vi "Teleop.vi"(10 "Match Info":T1={"Autonomous Elapsed Seconds"=0.0, "TeleOp Elapsed Seconds"=0.0, "Disabled Elapsed Seconds"=0.0, "Visited Autonomous"=FALSE, "Visited TeleOp"=FALSE, "Visited Disabled"=FALSE, "Autonomous Settings"={"Autonomous Style"=enum."Independent", "VI Refnum"=refnum}}, 11 "Call Context":T2) -> ()   [LabVIEW 2014]
doc: "This VI is called for each TeleOp packet received from the DS where the robot is not disabled. It is often used to read from the joysticks and update I/O or to update setpoints for timed control loops. It should complete and return within 20 milliseconds or it may miss DS packets."
uses:
  <vilib>/Rock Robotics/WPI/DriverStation/WPI_DriverStationDerivedRobotMode.ctl
  <vilib>/Rock Robotics/WPI/DriverStation/WPI_DriverStationMatch Info.ctl
  <vilib>/Rock Robotics/WPI/Solenoid/WPI_SolenoidValue.ctl
  <vilib>/Rock Robotics/WPI/RobotDrive/WPI_RobotDriveGetSetRefNum.vi
  <vilib>/Rock Robotics/WPI/Joystick/WPI_JoystickGetSetRefNum.vi
  <vilib>/Rock Robotics/Network Tables/SD Write Boolean Array.vi
  <vilib>/Rock Robotics/Network Tables/SD Write Numeric Array.vi
  <vilib>/Rock Robotics/WPI/Compressor/WPI_CompressorGetSetRefNum.vi
  <vilib>/Rock Robotics/WPI/Solenoid/WPI_SolenoidSetEnum.vi
  hhVI/hhVI.lvlib
panel:
  out "Compressor Running":bool
  out "Enabled":bool
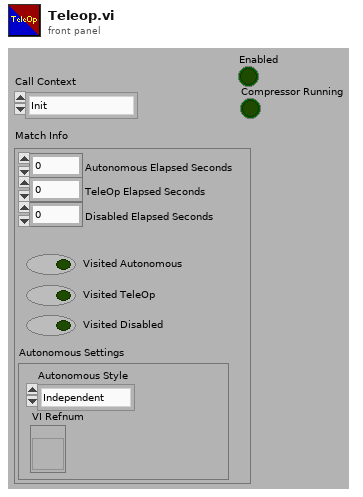
[diagram p1: front panel]
types:
  T1 = typedef "WPI_DriverStationMatch Info.ctl" = cluster{"Autonomous Elapsed Seconds":dbl, "TeleOp Elapsed Seconds":dbl, "Disabled Elapsed Seconds":dbl, "Visited Autonomous":bool, "Visited TeleOp":bool, "Visited Disabled":bool, "Autonomous Settings":cluster{"Autonomous Style":enum16{"Iterative", "Independent"}, "VI Refnum":refnum<vi>}}
  T2 = typedef "WPI_DriverStationDerivedRobotMode.ctl" = enum16{"Init", "Execute", "Stop"}
  T3 = typedef "WPI_RobotDriveDevRef.ctl" = cluster{"DevStatus":errorcluster, "Motors[]":T4[], "Square Inputs":bool, "Max Output":dbl}
  T4 = typedef "WPI_MotorControlDeviceRef.ctl" = cluster{"DeviceStatus":errorcluster, "Type":T5, "PWM":cluster{"Controller":T6, "PWM Channel":T7, "DeadBand":T8}, "CAN":cluster{"Device Number":u8, "Control Mode":T9, "Semaphore":T10, "Max Vout":dbl, "TalonSRX Control Mode":T11}, "Invert":bool, "TransformRef":T12, "InvTransformRef":T12}
  T5 = typedef "WPI_MotorControlType.ctl" = enum16{"PWM", "CAN", "CANTalonSRX"}
  T6 = typedef "FPGA_TypedefDigitalModule.ctl" = enum16{"Controller 1"}
  T7 = typedef "FPGA_DIOPWMChannel.ctl" = enum8{"PWM 0", "PWM 1", "PWM 2", "PWM 3", "PWM 4", "PWM 5", "PWM 6", "PWM 7", "PWM 8", "PWM 9", "PWM MXP 0", "PWM MXP 1", "PWM MXP 2", "PWM MXP 3", "PWM MXP 4", "PWM MXP 5", "PWM MXP 6", "PWM MXP 7", "PWM MXP 8", "PWM MXP 9", "Invalid"}
  T8 = typedef "WPI_PWMDeadband.ctl" = cluster{"Name":string, "maxPositivePwm":i32, "minPositivePwm":i32, "centerPwm":i32, "maxNegativePwm":i32, "minNegativePwm":i32, "angularRange":u16}
  T9 = typedef "WPI_CANJaguar_ControlMode.ctl" = enum8{"Percent VBus", "Current", "Speed", "Position", "Voltage"}
  T10 = typedef "Semaphore RefNum" = refnum<k1>
  T11 = typedef "WPI_CANTalonSRX_APIControlMode.ctl" = enum8{"Percent VBus", "Speed", "Position", "Slave", "Unchanged / Invalid"}
  T12 = typedef "WPI_PWMTransform_ConPane.ctl" = refnum<vi>
  T13 = typedef "WPI_JoystickDevRef.ctl" = cluster{"Device":T14}
  T14 = typedef "WPI_JoystickDeviceEnum.ctl" = enum16{"USB 0", "USB 1", "USB 2", "USB 3", "USB 4", "USB 5"}
  T15 = typedef "WPI_CompressorDevRef.ctl" = cluster{"DevStatus":errorcluster, "Pneumatics Control Module":u8}
  T16 = typedef "WPI_SolenoidDevRef.ctl" = cluster{"DevStatus":errorcluster, "Pneumatics Control Module":u8, "Forward Solenoid Channel":T17, "Reverse Solenoid Channel":T17}
  T17 = typedef "WPI_SolenoidChannel.ctl" = enum8{"Solenoid 0", "Solenoid 1", "Solenoid 2", "Solenoid 3", "Solenoid 4", "Solenoid 5", "Solenoid 6", "Solenoid 7", "Invalid"}
  T18 = typedef "WPI_SolenoidValue.ctl" = enum16{"Off", "On", "Forward", "Reverse"}
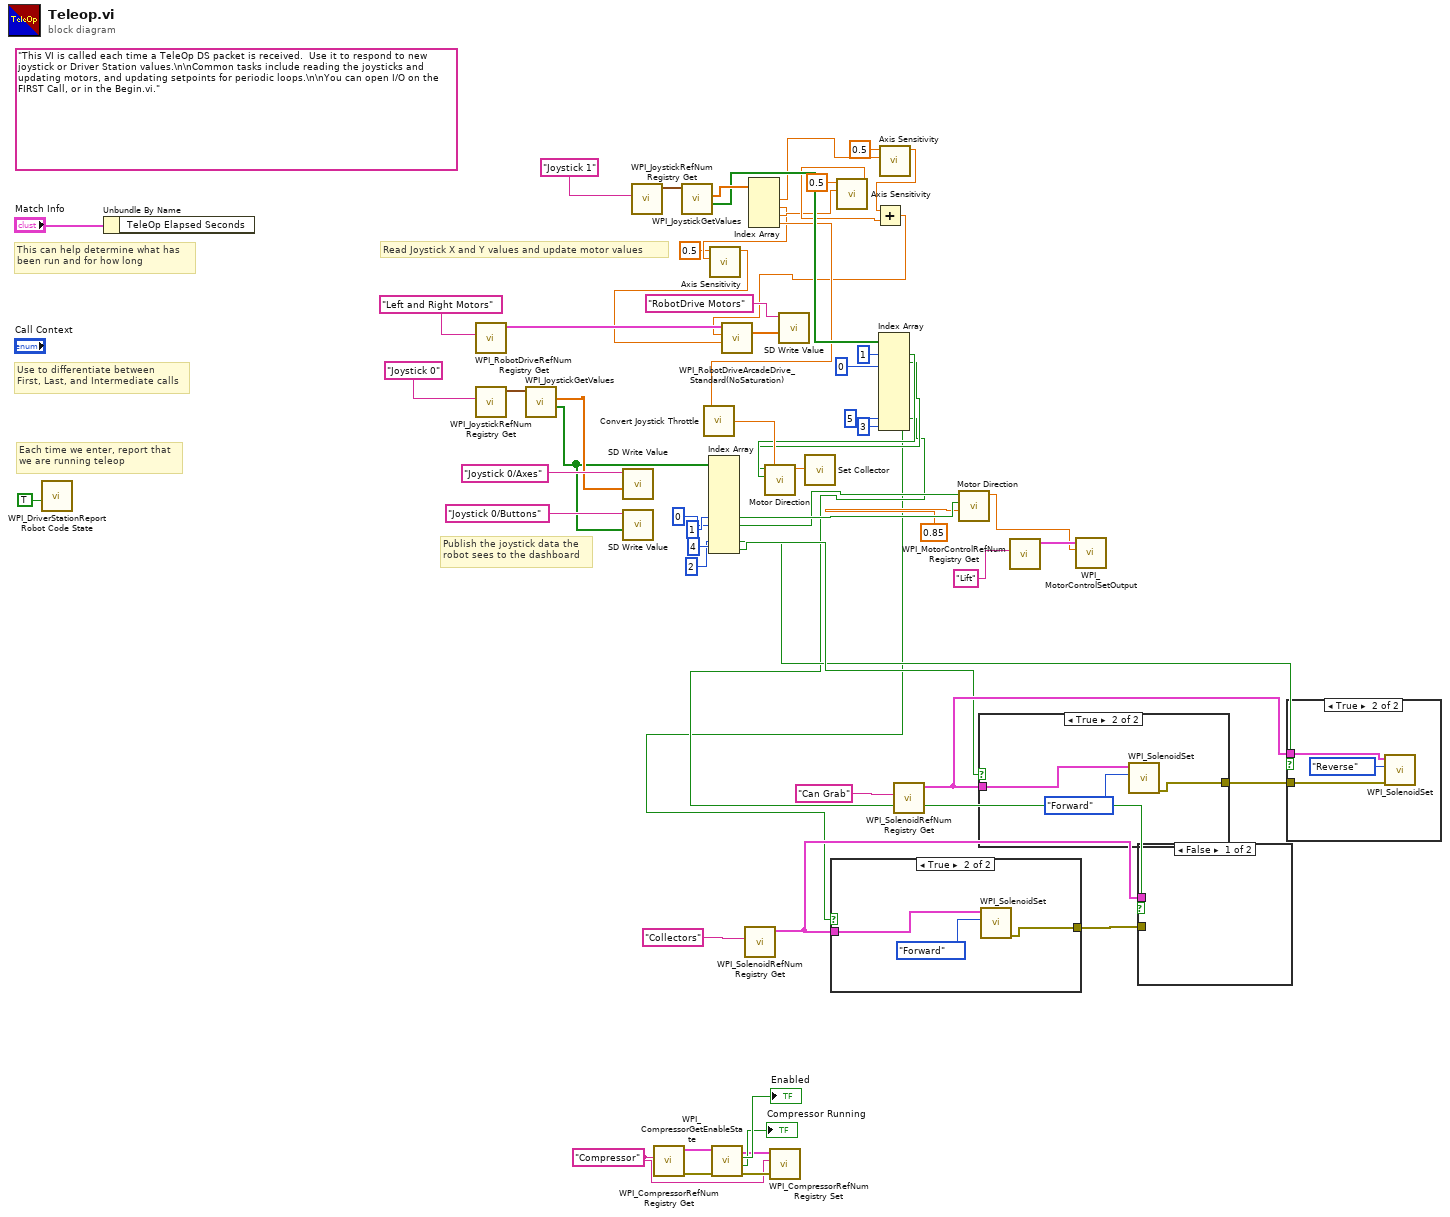
[diagram p0: block diagram]
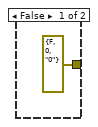
[diagram p3: hidden frame]
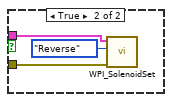
[diagram p4: hidden frame]
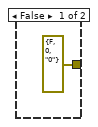
[diagram p5: hidden frame]
diagram:
  w42 = "Compressor" ("refnum name")
  (unwired) "This VI is called each time a TeleOp DS packet is received.  Use it to respond to new joystick or Driver Station values.\n\nCommon tasks include reading the joysticks and updating motors, and updating setpoints for periodic loops.\n\nYou can open I/O on the FIRST Call, or in the Begin.vi."
  # "Publish the joystick data the\nrobot sees to the dashboard"
  # "Each time we enter, report that\nwe are running teleop"
  # "Use to differentiate between\nFirst, Last, and Intermediate calls"
  # "This can help determine what has\nbeen run and for how long"
  # "Read Joystick X and Y values and update motor values"
  n1 = call <vilib>:"WPI_DriverStationReport Robot Code State.vi"("TeleOp"=TRUE ("Autonomous")) -> ()  [unwired: 10 in, 1 out]
  n2 = Unbundle By Name("Match Info") -> ()  [unwired: 1 out]
  n3 = call <vilib>:"WPI_RobotDriveRefNum Registry Get.vi"("refnum name"="Left and Right Motors") -> ("RobotDriveDevRef"=w60:T3)  [unwired: 1 in, 9 out]
  n4 = call <vilib>:"WPI_JoystickRefNum Registry Get.vi"("refnum name"="Joystick 0") -> ("JoystickDevRef"=w58:T13)  [unwired: 1 in, 9 out]
  n5 = call <vilib>:"WPI_JoystickGetValues.vi"("JoystickDevRef"=w58) -> ("Buttons"=w51:bool[], "Axes"=w52:dbl[])  [unwired: 6 in, 3 out]
  n6 = call-poly <vilib>:"SD Write Value.vi"("Numeric Array"=w52, "Name"="Joystick 0/Axes") -> ()  [unwired: 8 in, 2 out]
  n7 = call-poly <vilib>:"SD Write Value.vi"("Boolean Array"=w51, "Name"="Joystick 0/Buttons") -> ()  [unwired: 8 in, 2 out]
  n8 = call <vilib>:"WPI_JoystickRefNum Registry Get.vi"("refnum name"="Joystick 1") -> ("JoystickDevRef"=w38:T13)  [unwired: 1 in, 9 out]
  n9 = call <vilib>:"WPI_CompressorRefNum Registry Get.vi"("refnum name"=w42) -> ("error out"=w47:errorcluster, "CompressorDevRef"=w48:T15)  [unwired: 9 in]
  n10 = call <vilib>:"WPI_JoystickGetValues.vi"("JoystickDevRef"=w38) -> ("Buttons"=w20:bool[], "Axes"=w37:dbl[])  [unwired: 6 in, 3 out]
  n11 = Index Array(array=w51, index #6=1 ("index"), index #7=0 ("index"), index #9=2, index #10=4 ("index")) -> (element #6=w34:bool, element #7=w33:bool, element #9=w25:bool, element #10=w26:bool)  [unwired: 6 in, 6 out]
  n12 = call <vilib>:"WPI_CompressorGetEnableState.vi"("error in (no error)"=w47, "CompressorDevRef"=w48) -> ("error out"=w43:errorcluster, "Compressor Running"=→"Compressor Running":bool, "Enabled"=→"Enabled":bool, "CompressorDevRef"=w44:T15)  [unwired: 6 in]
  n13 = call <vilib>:"WPI_SolenoidRefNum Registry Get.vi"("refnum name"="Collectors") -> ("SolenoidDevRef"=w40:T16)  [unwired: 9 in, 1 out]
  n14 = Index Array(array=w37) -> (element #1=w6:dbl, element #2=w2:dbl, element #3=w4:dbl, element #4=w11:dbl)  [unwired: 4 in]
  n15 = call "Convert Joystick Throttle.vi"("Input"=w11) -> ("Output"=w22:dbl)
  n16 = call "Axis Sensitivity.vi"("Raw"=w2, "Sensitivity"=0.5) -> ("Output"=w3:dbl)  [unwired: 9 in]
  n17 = call <vilib>:"WPI_CompressorRefNum Registry Set.vi"("error in (no error)"=w43, "refnum name"=w42, "CompressorDevRef"=w44) -> ()  [unwired: 7 in, 2 out]
  n18 = call "Axis Sensitivity.vi"("Raw"=w4, "Sensitivity"=0.5) -> ("Output"=w5:dbl)  [unwired: 9 in]
  n19 = Index Array(array=w20, index #1=1 ("index"), index #2=0 ("index"), index #9=5 ("index"), index #10=3 ("index")) -> (element #1=w17:bool, element #2=w16:bool, element #9=w15:bool, element #10=w14:bool)  [unwired: 6 in, 6 out]
  n20 = call "Motor Direction.vi"("Speed"=w22, "Backwards"=w17, "Forward"=w16) -> ("Direction"=w50:dbl)  [unwired: 8 in]
  n21 = call "Set Collector.vi"("Speed"=w50) -> ()  [unwired: 11 in]
  n22 = case shown="True" w14 {
    tunnel: w40 -> [_ w64]
    tunnel: [errorcluster {"status"=FALSE, "code"=0, "source"="0"} ("error out") w65] -> w41
    frame False {
    }
    frame True {
      n23 = call-poly <vilib>:"WPI_SolenoidSet.vi"("Value"=WPI_SolenoidValue."Forward", "SolenoidDevRef"=w64) -> ("error out"=w65:errorcluster)  [unwired: 8 in, 1 out]
    }
  }
  n24 = call "Axis Sensitivity.vi"("Raw"=w6, "Sensitivity"=0.5) -> ("Output"=w8:dbl)  [unwired: 9 in]
  n25 = Add(x=w8, y=w5) -> (x+y=w10:dbl)
  n26 = call <vilib>:"WPI_RobotDriveArcadeDrive_Standard(NoSaturation).vi"("Y axis value"=w3, "X axis value"=w10, "RobotDriveDevRef"=w60) -> ("Motor Values"=w55:dbl[])  [unwired: 1 in, 7 out]
  n27 = call-poly <vilib>:"SD Write Value.vi"("Numeric Array"=w55, "Name"="RobotDrive Motors") -> ()  [unwired: 8 in, 2 out]
  n28 = call <vilib>:"WPI_SolenoidRefNum Registry Get.vi"("refnum name"="Can Grab") -> ("SolenoidDevRef"=w27:T16)  [unwired: 9 in, 1 out]
  n29 = call "Motor Direction.vi"("Speed"=0.85, "Backwards"=w34, "Forward"=w33) -> ("Direction"=w35:dbl)  [unwired: 8 in]
  n30 = case shown="True" w26 {
    tunnel: w27 -> [_ w68]
    tunnel: [errorcluster {"status"=FALSE, "code"=0, "source"="0"} ("error out") w69] -> w28
    frame False {
    }
    frame True {
      n31 = call-poly <vilib>:"WPI_SolenoidSet.vi"("Value"=WPI_SolenoidValue."Forward", "SolenoidDevRef"=w68) -> ("error out"=w69:errorcluster)  [unwired: 8 in, 1 out]
    }
  }
  n32 = call <vilib>:"WPI_MotorControlRefNum Registry Get.vi"("refnum name"="Lift") -> ("MotorControlDevRef"=w49:T4)  [unwired: 9 in, 1 out]
  n33 = call <vilib>:"WPI_MotorControlSetOutput.vi"("Output"=w35, "MotorControlDevRef"=w49) -> ()  [unwired: 7 in, 3 out]
  n34 = case shown="False" w15 {
    tunnel: w40 -> [_ w73]
    tunnel: w41 -> [_ w72]
    frame False {
    }
    frame True {
      n35 = call-poly <vilib>:"WPI_SolenoidSet.vi"("error in (no error)"=w72, "Value"=WPI_SolenoidValue."Reverse", "SolenoidDevRef"=w73) -> ()  [unwired: 7 in, 2 out]
    }
  }
  n36 = case shown="True" w25 {
    tunnel: w27 -> [_ w76]
    tunnel: w28 -> [_ w75]
    frame False {
    }
    frame True {
      n37 = call-poly <vilib>:"WPI_SolenoidSet.vi"("error in (no error)"=w75, "Value"=WPI_SolenoidValue."Reverse", "SolenoidDevRef"=w76) -> ()  [unwired: 7 in, 2 out]
    }
  }
